vi "ED_MRESET.vi"(4 "error in (no error)":errorcluster, 7 "connection ID":refnum<k5>) -> (0 "error out":errorcluster, 3 "connection ID out":refnum<k5>)   [LabVIEW 2020, in "CAENels EASY-DRIVER.lvlib"]
doc: "The MRESET block is used to perform a complete reset of the EASY-DRIVER module status register. This is needed, for example, to enable the channel output again after a fault condition has been fixed."
uses:
  CAENels EASY-DRIVER.lvlib
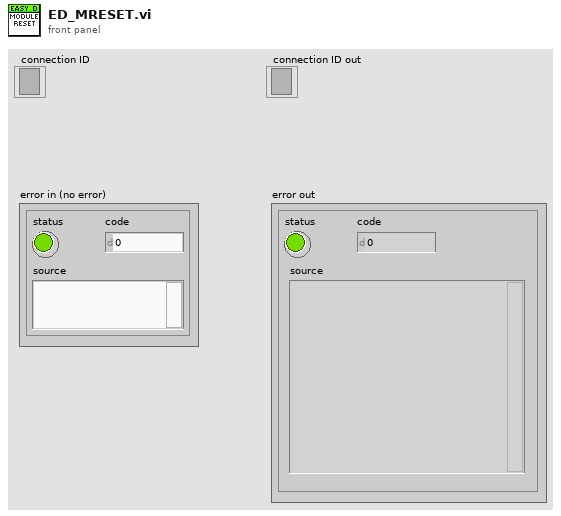
[diagram p1: front panel]
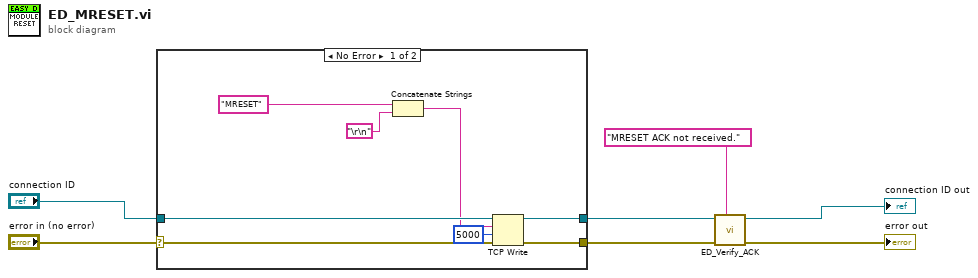
[diagram p0: block diagram]
diagram:
  n1 = case shown="No Error" "error in (no error)" {
    selector: "error in (no error)" -> [w15 w17]
    tunnel: [w14 w17] -> w5
    tunnel: [w13 w16] -> w3
    tunnel: "connection ID" -> [w12 w16]
    frame No Error {
      n2 = Concatenate Strings("MRESET" ("string (\"\")"), "\r\n") -> (w10:string)
      n3 = TCP Write(connection ID=w12, data in=w10, error in (no error)=w15, 9:5000 ("timeout ms (25000)")) -> (connection ID out=w13:refnum<k5>, error out=w14:errorcluster)  [unwired: 1 out]
    }
    frame Error {
    }
  }
  n4 = call "ED_Verify_ACK.vi"("error code description"="MRESET ACK not received.", "error in (no error)"=w5, "connection ID"=w3) -> ("error out"=→"error out":errorcluster, "connection ID out"=→"connection ID out":refnum<k5>)  [unwired: 5 in]
